vi "Assign Debugger to Actor.vi"(8 "error in (no error)":errorcluster, 10 "Actor index":i32, 11 "cRIO-CO2 in":refnum<class "cRIO-CO2.lvclass">) -> (0 "error out":errorcluster, 3 "cRIO-CO2 out":refnum<class "cRIO-CO2.lvclass">)   [LabVIEW 2015, in "cRIO-Carbondioxide.lvlib" / "cRIO-CO2.lvlib" / "cRIO-CO2.lvclass"]
uses:
  cRIO-CO2.lvclass
  cRIO-CO2.lvclass/cRIO-CO2.ctl
  <vilib>/ActorFramework/Actor/Actor.lvclass/Actor.ctl
  <vilib>/ActorFramework/Message Enqueuer/Message Enqueuer.lvclass/Message Enqueuer.ctl
  CO2 Actor Messages/Set Debugger Msg/Set Debugger Msg.lvclass/Set Debugger Msg.ctl
  <vilib>/ActorFramework/Actor/Read Self Enqueuer.vi
  <vilib>/ActorFramework/Message Enqueuer/Enqueue.vi
  <vilib>/ActorFramework/Message Enqueuer/Init from Existing Queue.vi
  <vilib>/ActorFramework/Message Priority Queue/Priority Enqueue.vi
  <vilib>/ActorFramework/Actor/Actor.lvclass
  <vilib>/ActorFramework/Message Enqueuer/Message Enqueuer.lvclass
  CO2 Actor Messages/Unset Debugger Msg/Unset Debugger Msg.lvclass
  CO2 Actor Messages/Set Debugger Msg/Set Debugger Msg.lvclass
  CO2 Actor/CO2 Actor.lvclass
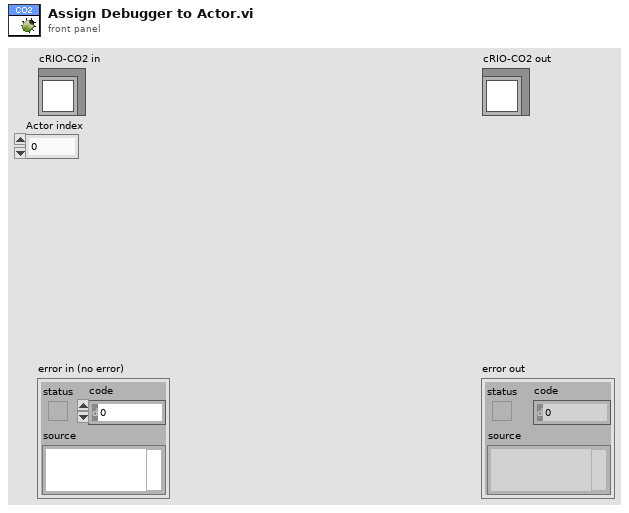
[diagram p1: front panel]
types:
  T1 = cluster{"dT/dt-Lower":dbl, "dT/dt":dbl, "dT/dt 2":dbl, "dT/dt 3":dbl, "dT/dt 4":dbl, "dT/dt-Lower 2":dbl, "dT/dt-Lower 3":dbl, "dT/dt 5":dbl}[]
  T2 = typedef "cRIO-Carbondioxide.lvlib/cRIO-CO2.lvlib/cRIO-CO2.lvclass/Debugger.ctl" = cluster{"Log Ref":refnum<vi>, "Debugger Graph Chart Ref":refnum<vi>, "Debug Rng Ref":refnum<vi>}
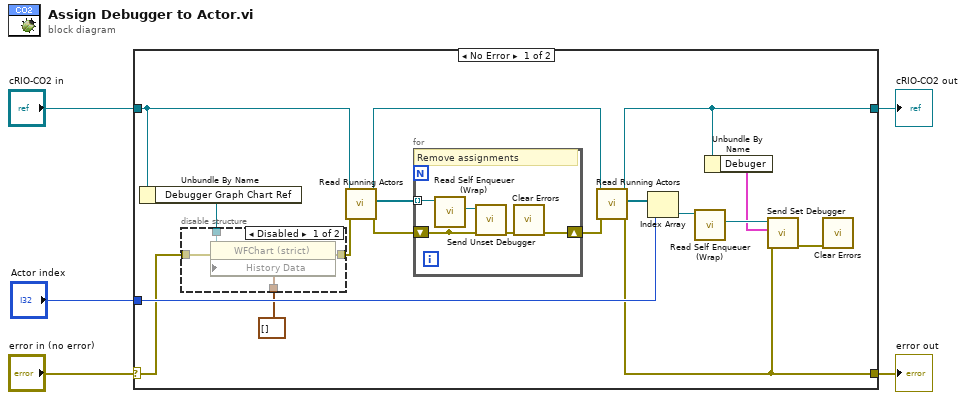
[diagram p0: block diagram]
diagram:
  n1 = case shown="No Error" "error in (no error)" {
    selector: "error in (no error)" -> [w6 w33]
    tunnel: [w14 w33] -> w4
    tunnel: [w18 w32] -> w2
    tunnel: "cRIO-CO2 in" -> [w10 w32]
    tunnel: "Actor index" -> [w20 _]
    frame No Error {
      n2 = Unbundle By Name(w10) -> ("Debugger Graph Chart Ref"=w9:refnum<vi>)
      n3 = disable-structure shown="Disabled" {
        disable-tunnel: w9 -> [w26 _]
        disable-tunnel: [w25 w27] -> w8
        disable-tunnel: T1 [] ("History Data") -> [w24 _]
        disable-tunnel: w6 -> [w23 w27]
        frame Disabled {
          n4 = property class="WFChart (strict)"(reference=w26, error in=w23, "History Data"=w24) -> (error out=w25:errorcluster)  [unwired: 1 out]
        }
        frame Enabled {
        }
      }
      n5 = call "Read Running Actors.vi"("error in (no error)"=w8, "cRIO-CO2 in"=w10) -> ("error out"=w12:errorcluster, "Running Actors"=w22:refnum<class "CO2 Actor.lvclass">[], "cRIO-CO2 out"=w19:refnum<class "cRIO-CO2.lvclass">)  [unwired: 7 in]
      n6 = for {
        tunnel: w22 -> [w30] mode=indexing
        shift-right: [w28] -> w11
        shift-left: w12 -> [w28]
        # "Remove assignments"
        n7 = call "Read Self Enqueuer (Wrap).vi"("CO2 Actor in"=w30) -> ("Actor Framework:Message Enqueuer"=w29:refnum<class "Message Enqueuer.lvclass">)  [unwired: 9 in, 1 out]
        n8 = call "Send Unset Debugger.vi"("error in (no error)"=w28, "Message Enqueuer"=w29) -> ("error out"=w31:errorcluster)  [unwired: 8 in, 1 out]
        n9 = call <vilib>:"Clear Errors.vi"("error in (no error)"=w31) -> ()  [unwired: 5 in, 2 out]
      }
      n10 = call "Read Running Actors.vi"("error in (no error)"=w11, "cRIO-CO2 in"=w19) -> ("error out"=w14:errorcluster, "Running Actors"=w21:refnum<class "CO2 Actor.lvclass">[], "cRIO-CO2 out"=w18:refnum<class "cRIO-CO2.lvclass">)  [unwired: 7 in]
      n11 = Index Array(array=w21, index=w20) -> (element=w16:refnum<class "CO2 Actor.lvclass">)
      n12 = call "Read Self Enqueuer (Wrap).vi"("CO2 Actor in"=w16) -> ("Actor Framework:Message Enqueuer"=w15:refnum<class "Message Enqueuer.lvclass">)  [unwired: 9 in, 1 out]
      n13 = Unbundle By Name(w18) -> ("Debuger"=w13:T2)
      n14 = call "Send Set Debugger.vi"("error in (no error)"=w14, "Debuger"=w13, "Message Enqueuer"=w15) -> ("error out"=w17:errorcluster)  [unwired: 7 in, 1 out]
      n15 = call <vilib>:"Clear Errors.vi"("error in (no error)"=w17) -> ()  [unwired: 5 in, 2 out]
    }
    frame Error {
    }
  }
  "error out" <- w4
  "cRIO-CO2 out" <- w2
